vi "activateAIDenoiser.vi"(0 "phConv in":u64, 11 "error in (no error)":errorcluster) -> (4 "phConv out":u64, 15 "error out":errorcluster)   [LabVIEW 2019]
uses:
  Convert.lvlib
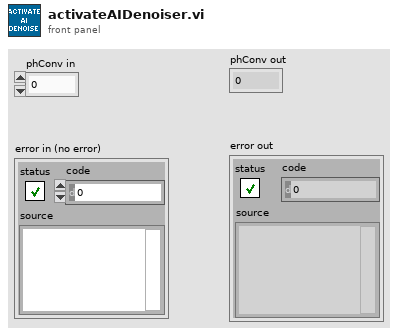
[diagram p1: front panel]
types:
  T1 = cluster{"PCO_Display":cluster{"wScale_minmax":u16, "iScale_maxmax":i32, "iScale_min":i32, "iScale_max":i32, "iColor_temp":i32, "iColor_tint":i32, "iColor_saturation":i32, "iColor_vibrance":i32, "iContrast":i32, "iGamma":i32, "iSRGB":i32, "pHistogramData":u64, "dwProcessingFlags":u32, "wProzValue4Min":u16, "wProzValue4Max":u16}, "PCO_Bayer":cluster{"iKernel":i32, "iColorMode":i32}, "PCO_Filter":cluster{"iMode":i32, "iType":i32, "iSharpen":i32}, "PCO_SensorInfo":cluster{"iConversionFactor":i32, "iDataBits":i32, "iSensorInfoBits":i32, "iDarkOffset":i32, "strColorCoeff":dbl[], "iCamNum":i32, "hCamera":u64}, "iData_Bits_Out":i32, "dwModeBitsDataOut":u32, "iGPU_Processing_mode":i32, "iConvertType":i32, "szConvertInfo":string, "dwConvertCAPS":u32}
  T2 = cluster{"iMode":i32, "iType":i32, "iSharpen":i32}
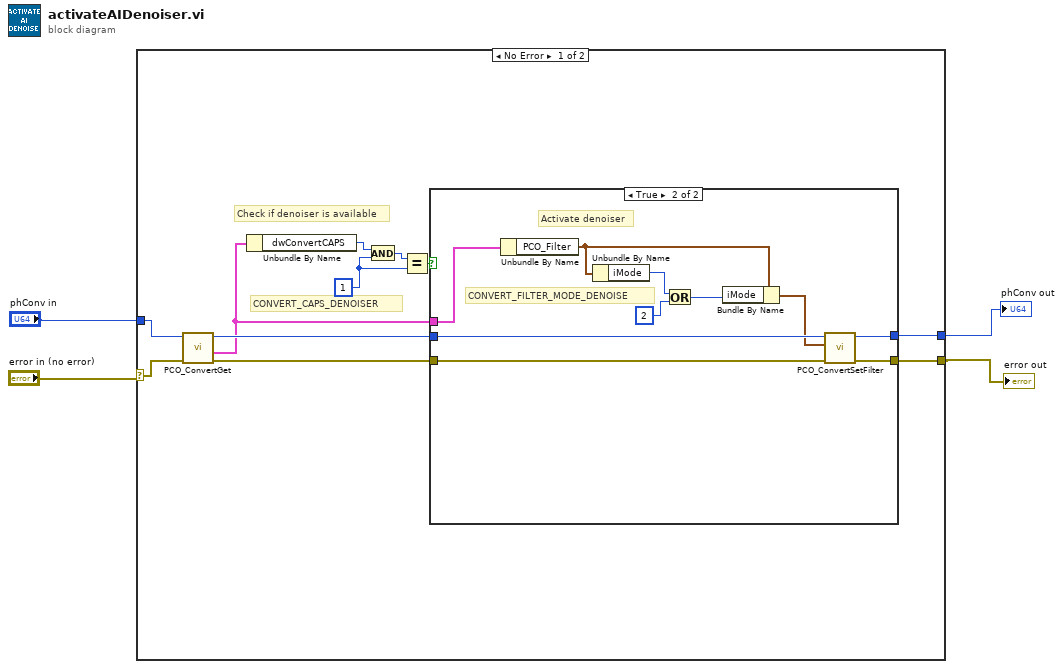
[diagram p0: block diagram]
diagram:
  n1 = case shown="No Error" "error in (no error)" {
    selector: "error in (no error)" -> [w14 w29]
    tunnel: "phConv in" -> [w15 w28]
    tunnel: [w6 w29] -> w1
    tunnel: [w7 w28] -> w2
    frame No Error {
      w11 = u32 1
      # "Check if denoiser is available"
      # "CONVERT_CAPS_DENOISER"
      n2 = call "PCO_ConvertGet.vi"("error in (no error)"=w14, "ph"=w15) -> ("error out"=w8:errorcluster, "strConvert"=w5:T1, "ph out"=w9:u64)  [unwired: 6 in, 1 out]
      n3 = Unbundle By Name(w5) -> ("dwConvertCAPS"=w13:u32)
      n4 = And(x=w13, y=w11) -> (x .and. y?=w12:u32)
      n5 = Equal?(x=w12, y=w11) -> (x = y?=w10:bool)
      n6 = case shown="True" w10 {
        tunnel: w9 -> [w17 w22]
        tunnel: w8 -> [w16 w21]
        tunnel: [w17 w19] -> w7
        tunnel: [w16 w20] -> w6
        tunnel: w5 -> [_ w27]
        frame False {
        }
        frame True {
          # "CONVERT_FILTER_MODE_DENOISE"
          # "Activate denoiser"
          n7 = Unbundle By Name(w27) -> ("PCO_Filter"=w26:T2)
          n8 = Unbundle By Name(w26) -> ("iMode"=w25:i32)
          n9 = Or(x=w25, y=2) -> (x .or. y?=w24:i32)
          n10 = Bundle By Name(cluster=w26, "iMode"=w24) -> (w18:T2)
          n11 = call "PCO_ConvertSetFilter.vi"("error in (no error)"=w21, "strFilter"=w18, "ph"=w22) -> ("error out"=w20:errorcluster, "ph out"=w19:u64)  [unwired: 6 in, 1 out]
        }
      }
    }
    frame Error {
    }
  }
  "error out" <- w1
  "phConv out" <- w2
